vi "GetPhysicalTriggerSettings.vi"(8 "error in (no error)":errorcluster, 11 "Highland T564 DDG in":refnum<class "Highland T564 DDG.lvclass">) -> (0 "error out":errorcluster, 3 "Highland T564 DDG out":refnum<class "Highland T564 DDG.lvclass">)   [LabVIEW 2020, in "Highland T564 DDG.lvclass"]
uses:
  Highland T564 DDG.lvclass
  C:/GEECS/Developers Version/source/Device Drivers/shared/MetaDriver_v1/MetaDriver_v1.lvclass
  Highland T564 DDG.lvclass/Highland T564 DDG.ctl
  Trigger.ctl
  Choice01.ctl
  TriggerImpedance.ctl
  TriggerSource.ctl
  T560Session.lvclass
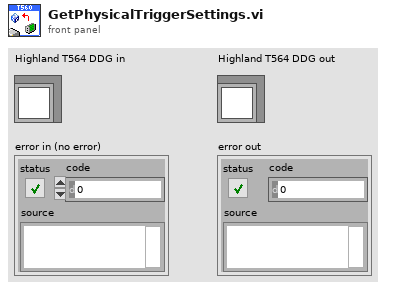
[diagram p1: front panel]
types:
  T1 = typedef "TriggerImpedance.ctl" = enum16{"10KOhm", "50Ohms"}
  T2 = typedef "TriggerSource.ctl" = enum16{"Rising", "Falling", "Internal 80MHz", "Internal DDS", "Remote", "Disabled"}
  T3 = cluster{"Trigger Divisor":string, "Trigger Level":string, "Impedance":T1, "TriggerSource":T2}
  T4 = typedef "Trigger.ctl" = cluster{"Divisor":T5, "Level":T5, "Impedance":T1, "Source":T2}
  T5 = typedef "Choice01.ctl" = cluster{"Value":dbl, "Min":dbl, "Max":dbl, "StepSize":dbl, "Tolerance":dbl, "ValueActual":dbl}
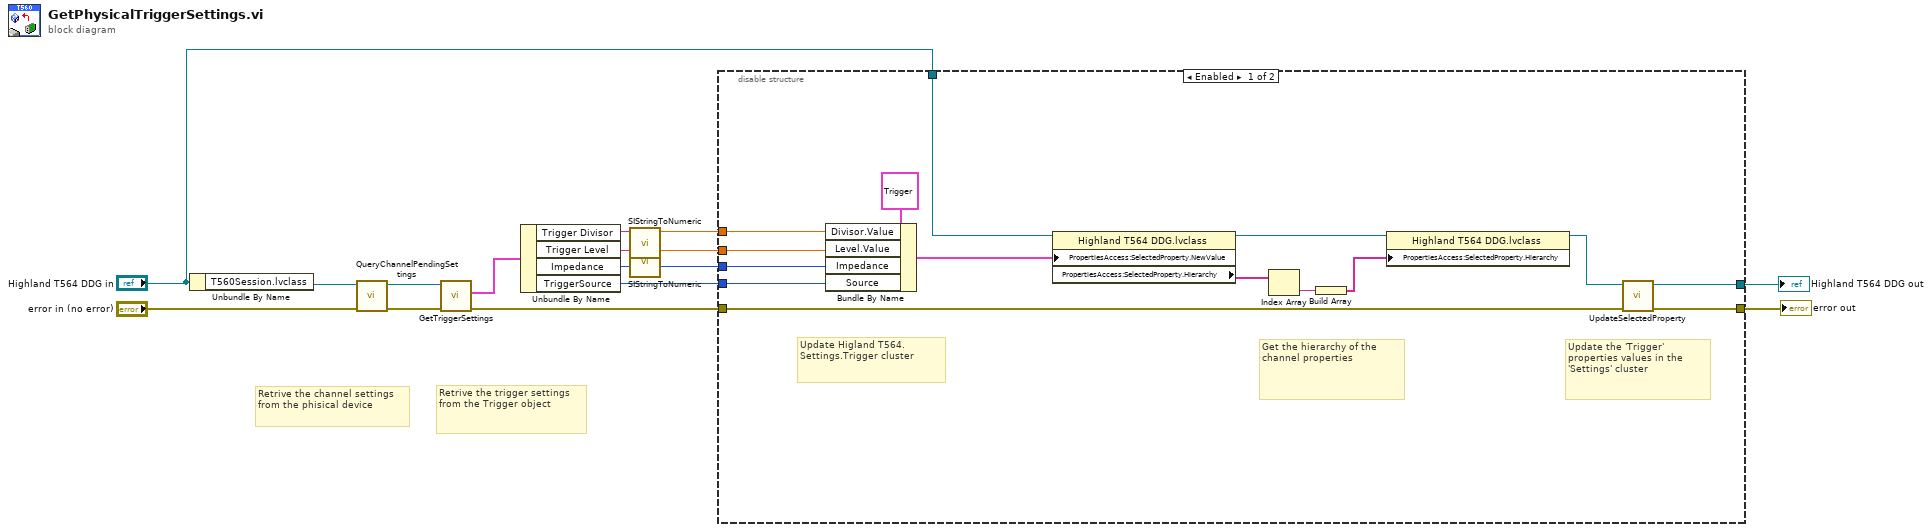
[diagram p0: block diagram]
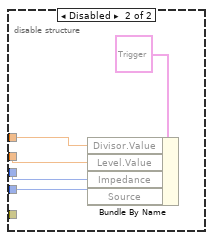
[diagram p2: hidden frame]
diagram:
  # "Retrive the channel settings from the phisical device"
  # "Retrive the trigger settings from the Trigger object"
  n1 = Unbundle By Name("Highland T564 DDG in") -> ("T560Session.lvclass"=w13:refnum<class "T560Session.lvclass">)
  n2 = call-dynamic "QueryChannelPendingSettings.vi"("error in"="error in (no error)", "T560Session in"=w13) -> ("error out"=w12:errorcluster, "T560Session out"=w10:refnum<class "T560Session.lvclass">)  [unwired: 8 in]
  n3 = call-dynamic "GetTriggerSettings.vi"("error in (no error)"=w12, "T560Session in"=w10) -> ("error out"=w2:errorcluster, "TriggerSettings"=w9:T3)  [unwired: 7 in, 1 out]
  n4 = Unbundle By Name(w9) -> ("Trigger Divisor"=w8:string, "Trigger Level"=w6:string, "Impedance"=w3:T1, "TriggerSource"=w4:T2)
  n5 = call "SIStringToNumeric.vi"("SI number"=w8) -> ("Number"=w7:dbl)  [unwired: 9 in, 1 out]
  n6 = call "SIStringToNumeric.vi"("SI number"=w6) -> ("Number"=w5:dbl)  [unwired: 9 in, 1 out]
  n7 = disable-structure shown="Enabled" {
    disable-tunnel: [w20 _] -> w15
    disable-tunnel: "Highland T564 DDG in" -> [w18 _]
    disable-tunnel: w7 -> [w30 w34]
    disable-tunnel: w5 -> [w29 w33]
    disable-tunnel: w4 -> [w28 w31]
    disable-tunnel: w3 -> [w27 w32]
    disable-tunnel: w2 -> [w16 _]
    disable-tunnel: [w21 _] -> w1
    frame Enabled {
      # "Update the 'Trigger' properties values in the 'Settings' cluster"
      # "Get the hierarchy of the channel properties"
      # "Update Higland T564.Settings.Trigger cluster"
      n8 = Bundle By Name(cluster=T4 {"Divisor"={"Value"=0.0, "Min"=0.0, "Max"=0.0, "StepSize"=0.0, "Tolerance"=0.0, "ValueActual"=0.0}, "Level"={"Value"=0.0, "Min"=0.0, "Max"=0.0, "StepSize"=0.0, "Tolerance"=0.0, "ValueActual"=0.0}, "Impedance"=enum."10KOhm", "Source"=enum."Rising"} ("Trigger"), "Divisor.Value"=w30, "Level.Value"=w29, "Impedance"=w27, "Source"=w28) -> (w17:T4)
      n9 = property class="Highland T564 DDG.lvclass"(reference=w18, "PropertiesAccess:SelectedProperty.NewValue"=w17) -> (reference out=w22:refnum<class "Highland T564 DDG.lvclass">, "PropertiesAccess:SelectedProperty.Hierarchy"=w24:string[])  [unwired: 1 in, 1 out]
      n10 = Index Array(array=w24) -> (element=w25:string)  [unwired: 1 in]
      n11 = Build Array(w25) -> (w26:string[])
      n12 = property class="Highland T564 DDG.lvclass"(reference=w22, "PropertiesAccess:SelectedProperty.Hierarchy"=w26) -> (reference out=w23:refnum<class "Highland T564 DDG.lvclass">)  [unwired: 1 in, 1 out]
      n13 = call-dynamic "UpdateSelectedProperty.vi"("error in (no error)"=w16, "Highland T564 DDG in"=w23) -> ("error out"=w21:errorcluster, "Highland T564 DDG out"=w20:refnum<class "Highland T564 DDG.lvclass">)  [unwired: 8 in]
    }
    frame Disabled {
      n14 = Bundle By Name(cluster=T4 {"Divisor"={"Value"=0.0, "Min"=0.0, "Max"=0.0, "StepSize"=0.0, "Tolerance"=0.0, "ValueActual"=0.0}, "Level"={"Value"=0.0, "Min"=0.0, "Max"=0.0, "StepSize"=0.0, "Tolerance"=0.0, "ValueActual"=0.0}, "Impedance"=enum."10KOhm", "Source"=enum."Rising"} ("Trigger"), "Divisor.Value"=w34, "Level.Value"=w33, "Impedance"=w32, "Source"=w31) -> ()  [unwired: 1 out]
    }
  }
  "Highland T564 DDG out" <- w15
  "error out" <- w1
